vi "DatabaseAPI-Query-SecondaryDb.vi"(7 "optional clause":string, 8 "error in (no error)":errorcluster, 9 "Columns":string, 10 "Table":string, 11 "Database-API in":refnum<class "Database-API.lvclass">) -> (0 "error out":errorcluster, 1 "columns":string[](array[string]), 2 "data":string[][](table), 3 "Database-API out":refnum<class "Database-API.lvclass">)   [LabVIEW 2014, in "Database-API.lvclass"]
uses:
  Database-API.lvclass
  Database-API.lvclass/Database-API.ctl
  <vilib>/addons/database/NI_Database_API.lvlib
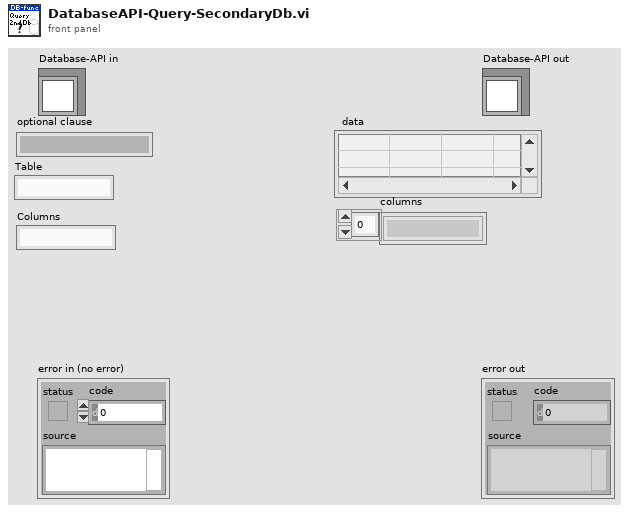
[diagram p1: front panel]
types:
  T1 = typedef "NI_Database_API.lvlib/Conn ObjectReference.ctl" = refnum<k1>
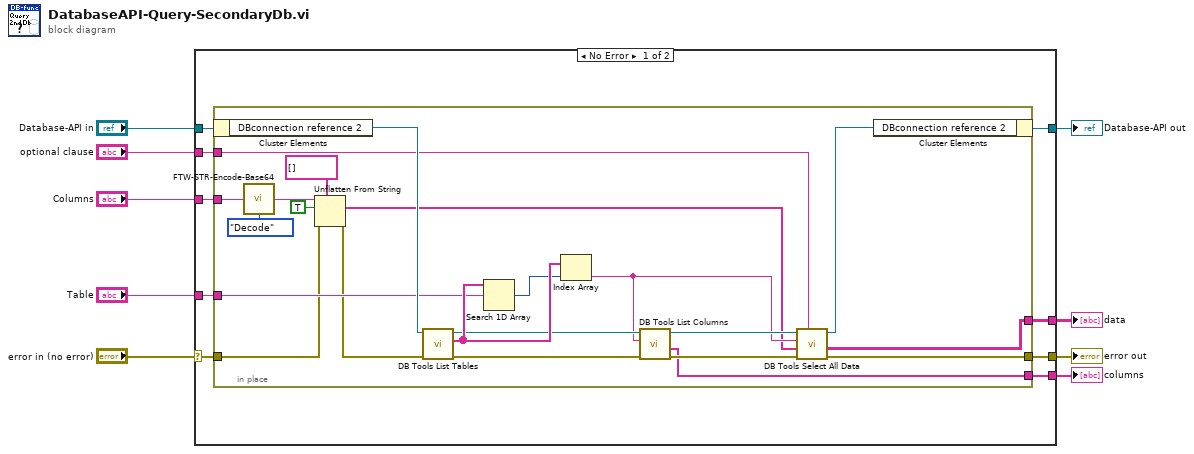
[diagram p0: block diagram]
diagram:
  n1 = case shown="No Error" "error in (no error)" {
    selector: "error in (no error)" -> [w18 w42]
    tunnel: [w16 w42] -> w8
    tunnel: [w15 w41] -> w6
    tunnel: "Database-API in" -> [w17 w41]
    tunnel: "Table" -> [w14 _]
    tunnel: "optional clause" -> [w13 _]
    tunnel: "Columns" -> [w12 _]
    tunnel: [w11 _] -> w2
    tunnel: [w10 _] -> w1
    frame No Error {
      n2 = in-place {
        in-place-border: w18 -> [w27]
        in-place-border: [w38] -> w16
        in-place-border: w14 -> [w30]
        in-place-border: w13 -> [w29]
        in-place-border: w12 -> [w22]
        in-place-border: [w24] -> w11
        in-place-border: [w23] -> w10
        n3 = in-place-cluster #1(w17) -> ("DBconnection reference 2"=w40:T1)
        n4 = call "FTW-STR-Encode-Base64.vi"("Input"=w22, "Direction"=enum16{"Encode", "Decode"}."Decode") -> ("Output"=w20:string)
        n5 = Unflatten From String(type=string[] [] ("Columns"), binary string=w20, data includes array or string size? (T)=TRUE, error in (no error)=w27) -> (value=w25:string[], error out=w26:errorcluster)  [unwired: 1 in, 1 out]
        n6 = call <vilib>:"DB Tools List Tables.vi"("error in (no error)"=w26, "connection reference"=w40) -> ("error out"=w34:errorcluster, "tables"=w37:string[], "connection reference out"=w35:T1)  [unwired: 3 in]
        n7 = Search 1D Array(1D array=w37, element=w30) -> (index of element=w36:i32)  [unwired: 1 in]
        n8 = Index Array(array=w37, index=w36) -> (element=w32:string)
        n9 = call <vilib>:"DB Tools List Columns.vi"("error in (no error)"=w34, "table"=w32, "connection reference"=w35) -> ("error out"=w31:errorcluster, "columns"=w23:string[], "connection reference out"=w33:T1)  [unwired: 1 in, 1 out]
        n10 = call <vilib>:"DB Tools Select All Data.vi"("optional clause"=w29, "error in (no error)"=w31, "columns"=w25, "table"=w32, "connection reference"=w33) -> ("error out"=w38:errorcluster, "data"=w24:string[][], "connection reference out"=w39:T1)  [unwired: 1 in]
        n11 = in-place-cluster #1("DBconnection reference 2"=w39) -> (w15:refnum<class "Database-API.lvclass">)
      }
    }
    frame Error {
    }
  }
  "error out" <- w8
  "Database-API out" <- w6
  "data" <- w2
  "columns" <- w1
